vi "uintArrayLCM.vi"(8 "Error in (no error)":errorcluster, 11 "Uint array in":refnum<class "UintClass.lvclass">[](array[class])) -> (0 "Error out":errorcluster, 1 "Timing":u32, 3 "LCM(Uint array)":refnum<class "UintClass.lvclass">)   [LabVIEW 2011, in "UintClass.lvclass"]
uses:
  UintClass.lvclass
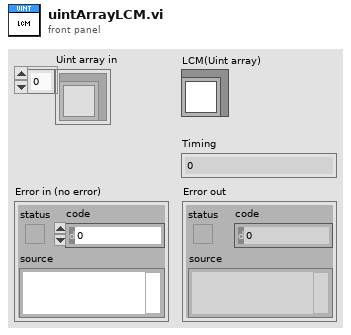
[diagram p1: front panel]
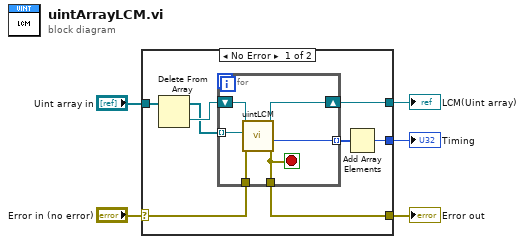
[diagram p0: block diagram]
diagram:
  n1 = case shown="No Error" "Error in (no error)" {
    selector: "Error in (no error)" -> [w13 w20]
    tunnel: "Uint array in" -> [w8 _]
    tunnel: [w12 w20] -> w3
    tunnel: [w11 _] -> w2
    tunnel: [w9 _] -> w1
    frame No Error {
      n2 = Delete From Array(array=w8) -> (deleted portion=w7:refnum<class "UintClass.lvclass">, array with subset deleted=w6:refnum<class "UintClass.lvclass">[])  [unwired: 2 in]
      n3 = for {
        tunnel: w6 -> [w19] mode=indexing
        shift-right: [w17] -> w11
        shift-left: w7 -> [w18]
        tunnel: [w14] -> w10 mode=indexing
        tunnel: w13 -> [w16]
        tunnel: [w15] -> w12
        stop <- w15 stop-if-true
        n4 = call "uintLCM.vi"("Error in (no error)"=w16, "Int2 in"=w19, "Int1 in"=w18) -> ("Error out"=w15:errorcluster, "Timing"=w14:u32, "LCM(Int1,Int2)"=w17:refnum<class "UintClass.lvclass">)  [unwired: 6 in]
      }
      n5 = Add Array Elements(numeric array=w10) -> (sum=w9:u32)
    }
    frame Error {
    }
  }
  "Error out" <- w3
  "LCM(Uint array)" <- w2
  "Timing" <- w1
